vi "Get Alias Mappings from Channel ID.vi"(8 "error in (no error)":errorcluster, 10 "Modules and Connections":T1[](array[typedef])=[{" Module Path"="", "Short Module Path"="", "Product Name"="", "Possible Connections"=[], "Missing"=FALSE}, {" Module Path"="", "Short Module Path"="", "Product Name"="", "Possible Connections"=[], "Missing"=FALSE}], 11 "Routing Channel Ref in":T4 format="%.0x") -> (0 "error out":errorcluster, 1 "Mappings by Module UI":T3[](array[typedef]), 2 "Alias Mappings UI":T5[](array[typedef]), 3 "Routing Channel Ref out":T4 format="%.0x")   [LabVIEW 2020, in "Routing and Faulting System Explorer.lvlib"]
uses:
  Routing and Faulting System Explorer.lvlib
  Shared/Alias Mapping.ctl
  Shared/Alias Endpoint.ctl
  <vilib>/NI VeriStand/Custom Device API/Custom Device Item Ref.ctl
  Alias Map by Module.ctl
  Possible Connections.ctl
  Shared/Routing and Faulting Hardware API/Types/Possible Connections for Endpoint.ctl
  Scripting/Routing and Faulting Scripting.lvlib
  <vilib>/NI VeriStand/Custom Device API/Custom Device API.lvlib
  Shared/Routing and Faulting Shared.lvlib
  Shared/Routing and Faulting Hardware API/Routing and Faulting Hardware API.lvlib
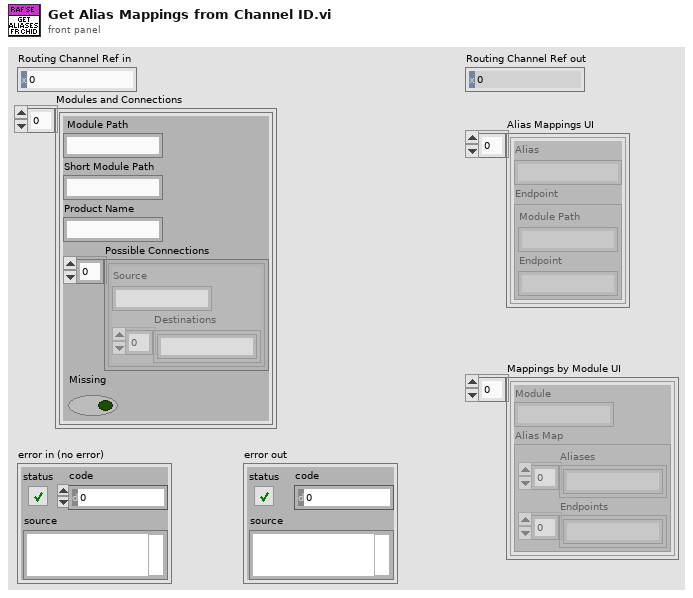
[diagram p1: front panel]
types:
  T1 = typedef "Routing and Faulting System Explorer.lvlib/Possible Connections.ctl" = cluster{" Module Path":string, "Short Module Path":string, "Product Name":string, "Possible Connections":T2[], "Missing":bool}
  T2 = typedef "Routing and Faulting Hardware API.lvlib/Possible Connections for Endpoint.ctl" = cluster{"Source":string, "Destinations":string[]}
  T3 = typedef "Routing and Faulting System Explorer.lvlib/Alias Map by Module.ctl" = cluster{"Module":string, "Alias Map":cluster{"Aliases":string[], "Endpoints":string[]}}
  T4 = typedef "Custom Device API.lvlib/Custom Device Item Ref.ctl" = u64
  T5 = typedef "Routing and Faulting Shared.lvlib/Alias Mapping.ctl" = cluster{"Alias":string, "Endpoint":T6}
  T6 = typedef "Routing and Faulting Shared.lvlib/Alias Endpoint.ctl" = cluster{"Module Path":string, "Endpoint":string}
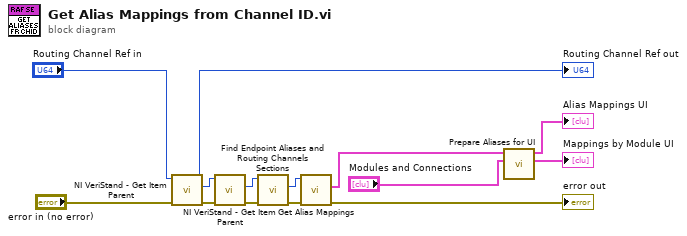
[diagram p0: block diagram]
diagram:
  n1 = call <vilib>:"NI VeriStand - Get Item Parent.vi"("error in (no error)"="error in (no error)", "Item Ref in"="Routing Channel Ref in") -> ("error out"=w10:errorcluster, "Parent Ref"=w11:T4, "Item Ref out"=→"Routing Channel Ref out":T4)  [unwired: 6 in, 1 out]
  n2 = call <vilib>:"NI VeriStand - Get Item Parent.vi"("error in (no error)"=w10, "Item Ref in"=w11) -> ("error out"=w13:errorcluster, "Parent Ref"=w12:T4)  [unwired: 6 in, 2 out]
  n3 = call "Find Endpoint Aliases and Routing Channels Sections.vi"("error in"=w13, "routing and faulting custom device in"=w12) -> ("error out"=w9:errorcluster, "endpoint aliases"=w8:T4)  [unwired: 6 in, 2 out]
  n4 = call "Get Alias Mappings.vi"("error in"=w9, "endpoint aliases in"=w8) -> ("error out"=→"error out":errorcluster, "alias mappings"=w3:T5[])  [unwired: 7 in, 1 out]
  n5 = call "Prepare Aliases for UI.vi"("Modules and Connections"="Modules and Connections", "Alias Mappings"=w3) -> ("Mappings by Module UI"=→"Mappings by Module UI":T3[], "Alias Mappings UI"=→"Alias Mappings UI":T5[])  [unwired: 8 in]
